vi "Change State.vi"(0 "TLB' data in":refnum<class "Springboard TLB`.lvclass">, 11 "error in":errorcluster) -> (4 "TLB' data out":refnum<class "Springboard TLB`.lvclass">, 15 "error out":errorcluster)   [LabVIEW 2018, in "Springboard TLB`.lvlib" / "Springboard TLB`.lvclass"]
doc: "Change system state.\n\n<B>Input Parameters</B>\n\n<B>TLB' data in</B> is the templates' private data.\n\n<B>error in</B> describes error conditions that occur before this node runs. This input provides standard error in functionality.\n\n<B>Output Parameters</B>\n\n<B>TLB' data out</B> is the templates' private data.\n\n<B>error out</B> contains error information. This output provides standard error out functionality."
uses:
  Springboard TLB`.lvclass
  Springboard TLB`.lvlib
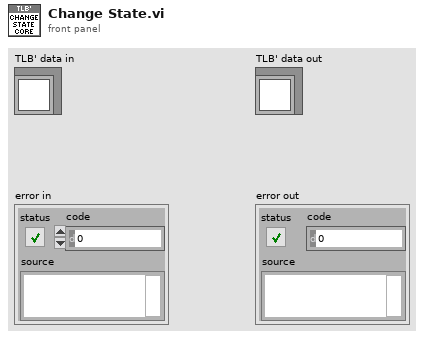
[diagram p1: front panel]
types:
  T1 = typedef "Springboard TLB`.lvlib/Springboard TLB`.lvclass/State.ctl" = enum16{"<Startup>", "Idle", "Creating", "<Shutdown>", "<Error>"}
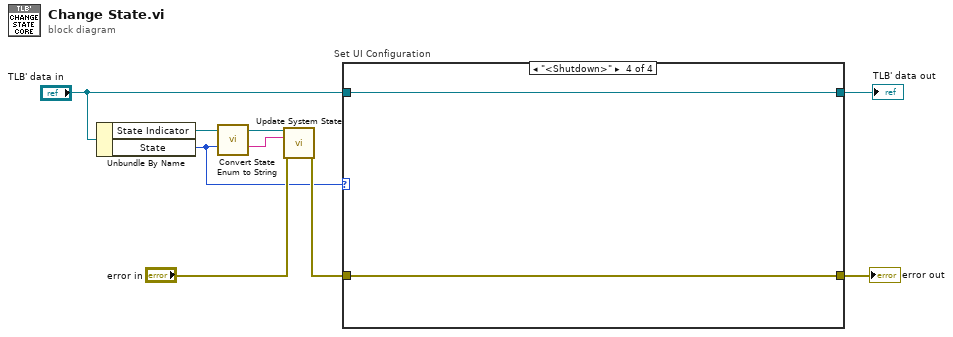
[diagram p0: block diagram]
diagram:
  n1 = Unbundle By Name("TLB' data in") -> ("State Indicator"=w5:refnum<user-event>, "State"=w1:T1)
  n2 = call "Convert State Enum to String.vi"("state in"=w1) -> ("state out"=w4:string)  [unwired: 13 in, 1 out]
  n3 = call "Update System State.vi"("State Indicator"=w5, "system state message"=w4, "error in"="error in") -> ("error out"=w2:errorcluster)  [unwired: 12 in]
  n4 = case "Set UI Configuration" shown="\"<Shutdown>\"" w1 {
    tunnel: [w9 w12 w13 w16] -> w7
    tunnel: w2 -> [w9 w12 w13 w16]
    tunnel: [w10 w11 w14 w15] -> w8
    tunnel: "TLB' data in" -> [w10 w11 w14 w15]
    frame "<Startup>" {
    }
    frame "Idle" {
    }
    frame "<Error>" {
    }
    frame "<Shutdown>" {
    }
  }
  "TLB' data out" <- w8
  "error out" <- w7
